vi "mockbusTesting.vi"() -> ()   [LabVIEW 2016]
uses:
  Common_FPGA_HealthAndStatus/DataTypes/HealthAndStatusSettings.ctl
  Common_FPGA_Modbus/DataTypes/ModbusPortSettings.ctl
  Common_FPGA_Timestamp/DataTypes/TimestampSettings.ctl
  FPGAMockHPILC/DataTypes/MockHPILCSettings.ctl
  <vilib>/rvi/Emulation/niFpgaGetClockAttributes.vi
  <vilib>/rvi/Emulation/niFpgaSctlEmulationGetInTimedLoop.vi
  <vilib>/rvi/Emulation/niFpgaEmulationReportErrorSimple.vi
  <vilib>/rvi/eio/common/nirviEmuTemplateMethod_errors.vi
  <vilib>/rvi/Emulation/niFpgaCriticalErrorInLSC.vi
  <vilib>/rvi/Emulation/niFpgaEmulationIsFPGAContextNoSignature.vi
  <vilib>/rvi/DataTransferAndStorage/Container/Common/niFpgaContainerGetUniqueNameForEmu.vi
  <vilib>/rvi/Memory/Memory_Emulation/niFpgaMemoryEmulationCacheClearOnFirstRun.vi
  <vilib>/rvi/Memory/Memory_Emulation/nirvimemoryEmulationManagerCache_MakeExclusive.vi
  <vilib>/rvi/Memory/Memory_Emulation/niFpgaMemoryEmulationValidateCache.vi
  <vilib>/rvi/Memory/Memory_Emulation/nirvimemoryEmulationManagerCache_InsertValue.vi
  <vilib>/Utility/error.llb/Clear Errors.vi
  <vilib>/rvi/Memory/Memory_Emulation/nirvimemoryEmulationManagerCache_ReleaseExclusive.vi
  <vilib>/rvi/Memory/Memory_Emulation/nirvimemoryEmulationManagerCache_GetValue.vi
  <vilib>/rvi/Memory/Memory_Emulation/nirvimemoryEmulationManagerCache_SetValue.vi
  <vilib>/rvi/Emulation/niFpgaProcessEmulError.vi
  <vilib>/eio/EIOMethodNode/EIOMethodNode.xnode
  <vilib>/rvi/DataTransferAndStorage/Container/XNode/niFpgaContainer.xnode
  <vilib>/rvi/DataTransferAndStorage/Register/Emulation/niFpgaRegisterEmulation.vi
  Common_FPGA_HealthAndStatus/FPGAHealthAndStatus.lvlib
  Common_FPGA_Modbus/FPGAModbus.lvlib
  Common_FPGA_Timestamp/FPGATimestamp.lvlib
  FPGAMockHPILC/FPGAMockHPILC.lvlib
panel:
  in  "Trigger":bool
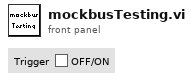
[diagram p1: front panel]
types:
  T1 = typedef "FPGAMockHPILC.lvlib/MockHPILCSettings.ctl" = cluster{"ModbusRxDataFIFO":refnum<k21>, "ModbusTxDataFIFO":refnum<k21>, "BufferUpdateFIFO":refnum<k21>, "Code17Memory":refnum<k21>, "Code18Memory":refnum<k21>, "Code65Memory":refnum<k21>, "Code66Memory":refnum<k21>, "Code67Memory":refnum<k21>, "Code72Memory":refnum<k21>, "Code80Memory":refnum<k21>, "Code110Memory":refnum<k21>, "CRCDataFIFO":refnum<k21>, "CRCCalculateFIFO":refnum<k21>, "CRCFIFO":refnum<k21>}
  T2 = typedef "FPGAModbus.lvlib/ModbusPortSettings.ctl" = cluster{"TxPort":refnum<k21>, "TxDataFIFO":refnum<k21>, "TxInternalDataFIFO":refnum<k21>, "TxHealthAndStatusFIFO":refnum<k21>, "RxPort":refnum<k21>, "RxDataFIFO":refnum<k21>, "RxHealthAndStatusFIFO":refnum<k21>, "BaseHealthAndStatusAddress":u32, "WaitForRxFrameRegister":refnum<k21>, "IRQAddress":u8, "TriggerIRQRegister":refnum<k21>, "InternalHealthAndStatusFIFO":refnum<k21>, "SoftwareControlledTrigger":refnum<k21>, "TimestampRegister":refnum<k21>, "TxTimestampFIFO":refnum<k21>}
  T3 = typedef "FPGATimestamp.lvlib/TimestampSettings.ctl" = cluster{"TimeRegister":refnum<k21>, "TimeSource":refnum<k21>, "IterationsPerMicrosecond":i16, "UpdateFIFO":refnum<k21>}
  T4 = typedef "FPGAHealthAndStatus.lvlib/HealthAndStatusSettings.ctl" = cluster{"InternalHealthAndStatusFIFO":refnum<k21>, "HealthAndStatusQueryFIFO":refnum<k21>, "HealthAndStatusResponseFIFO":refnum<k21>, "HealthAndStatusMemory":refnum<k21>, "MemorySize":i32}
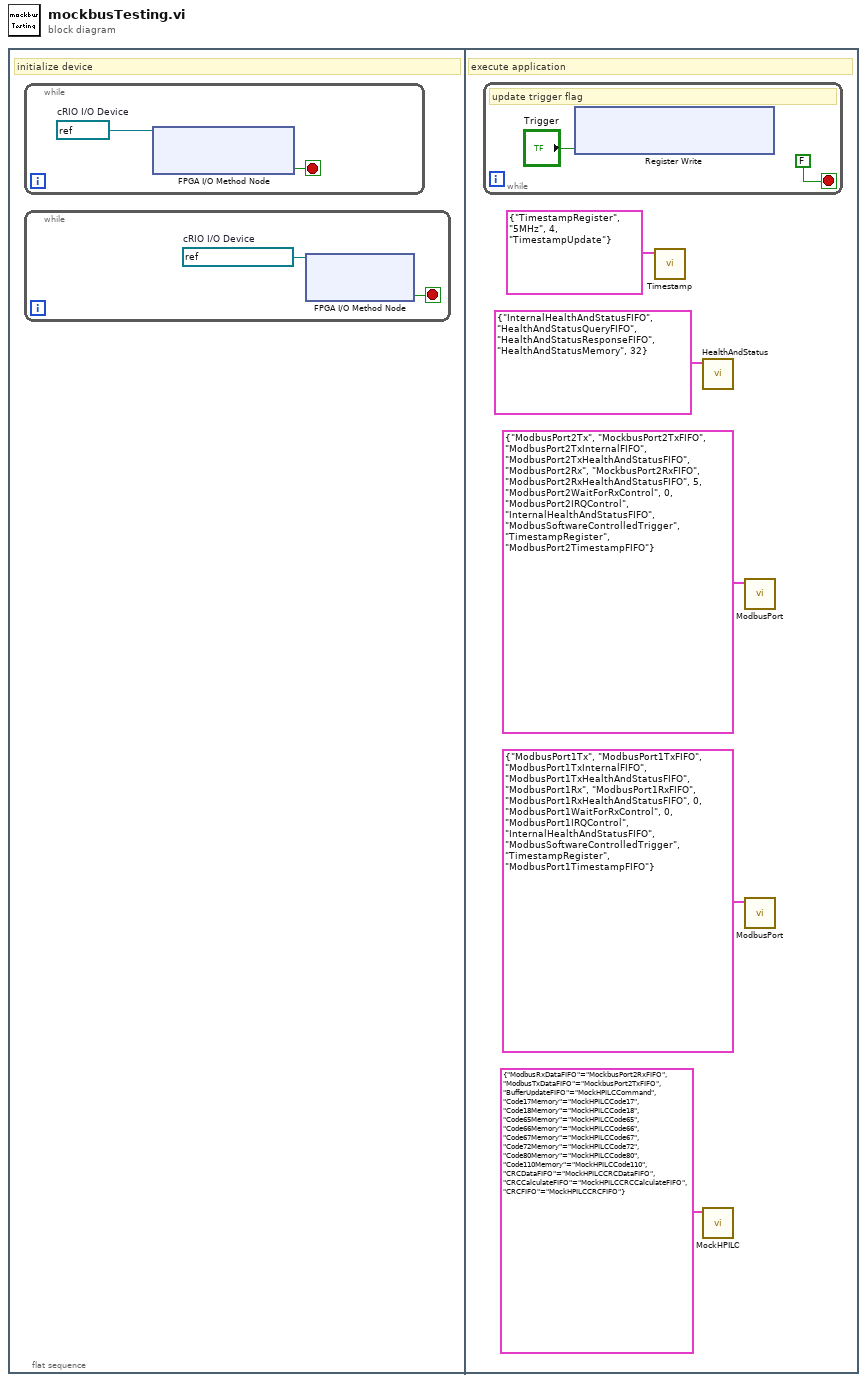
[diagram p0: block diagram]
diagram:
  n1 = flat-sequence {
    frame #0 {
      # "initialize device"
      n2 = while {
        stop <- w1 stop-if-true
        w2 = refnum<k21> "Sync"  # cRIO I/O Device
        n3 = xnode "FPGA I/O Method Node"("FPGA I/O In"=w2) -> ("Clock Running"=w1:bool)  [unwired: 1 out]
      }
      n4 = while {
        stop <- w3 stop-if-true
        w4 = refnum<k21> "ModbusPort1-4"  # cRIO I/O Device
        n5 = xnode "FPGA I/O Method Node"("FPGA I/O In"=w4) -> ("Ready"=w3:bool)  [unwired: 1 out]
      }
    }
    frame #1 {
      # "execute application"
      n6 = while {
        stop <- FALSE stop-if-true
        # "update trigger flag"
        n7 = xnode ("Register Write")("Data"="Trigger") -> ()  [unwired: 1 in, 1 out]
      }
      n8 = call "Timestamp.vi"("TimestampSettings"=T3 {"TimeRegister"="TimestampRegister", "TimeSource"="5MHz", "IterationsPerMicrosecond"=4, "UpdateFIFO"="TimestampUpdate"}) -> ()  [unwired: 11 in]
      n9 = call "HealthAndStatus.vi"("HealthAndStatusSettings"=T4 {"InternalHealthAndStatusFIFO"="InternalHealthAndStatusFIFO", "HealthAndStatusQueryFIFO"="HealthAndStatusQueryFIFO", "HealthAndStatusResponseFIFO"="HealthAndStatusResponseFIFO", "HealthAndStatusMemory"="HealthAndStatusMemory", "MemorySize"=32}) -> ()  [unwired: 11 in]
      n10 = call "MockHPILC.vi"("MockHPILCSettings"=T1 {"ModbusRxDataFIFO"="MockbusPort2RxFIFO", "ModbusTxDataFIFO"="MockbusPort2TxFIFO", "BufferUpdateFIFO"="MockHPILCCommand", "Code17Memory"="MockHPILCCode17", "Code18Memory"="MockHPILCCode18", "Code65Memory"="MockHPILCCode65", "Code66Memory"="MockHPILCCode66", "Code67Memory"="MockHPILCCode67", "Code72Memory"="MockHPILCCode72", "Code80Memory"="MockHPILCCode80", "Code110Memory"="MockHPILCCode110", "CRCDataFIFO"="MockHPILCCRCDataFIFO", "CRCCalculateFIFO"="MockHPILCCRCCalculateFIFO", "CRCFIFO"="MockHPILCCRCFIFO"}) -> ()  [unwired: 11 in]
      n11 = call "ModbusPort.vi"("ModbusPortSettings"=T2 {"TxPort"="ModbusPort2Tx", "TxDataFIFO"="MockbusPort2TxFIFO", "TxInternalDataFIFO"="ModbusPort2TxInternalFIFO", "TxHealthAndStatusFIFO"="ModbusPort2TxHealthAndStatusFIFO", "RxPort"="ModbusPort2Rx", "RxDataFIFO"="MockbusPort2RxFIFO", "RxHealthAndStatusFIFO"="ModbusPort2RxHealthAndStatusFIFO", "BaseHealthAndStatusAddress"=5, "WaitForRxFrameRegister"="ModbusPort2WaitForRxControl", "IRQAddress"=0, "TriggerIRQRegister"="ModbusPort2IRQControl", "InternalHealthAndStatusFIFO"="InternalHealthAndStatusFIFO", "SoftwareControlledTrigger"="ModbusSoftwareControlledTrigger", "TimestampRegister"="TimestampRegister", "TxTimestampFIFO"="ModbusPort2TimestampFIFO"}) -> ()  [unwired: 10 in]
      n12 = call "ModbusPort.vi"("ModbusPortSettings"=T2 {"TxPort"="ModbusPort1Tx", "TxDataFIFO"="ModbusPort1TxFIFO", "TxInternalDataFIFO"="ModbusPort1TxInternalFIFO", "TxHealthAndStatusFIFO"="ModbusPort1TxHealthAndStatusFIFO", "RxPort"="ModbusPort1Rx", "RxDataFIFO"="ModbusPort1RxFIFO", "RxHealthAndStatusFIFO"="ModbusPort1RxHealthAndStatusFIFO", "BaseHealthAndStatusAddress"=0, "WaitForRxFrameRegister"="ModbusPort1WaitForRxControl", "IRQAddress"=0, "TriggerIRQRegister"="ModbusPort1IRQControl", "InternalHealthAndStatusFIFO"="InternalHealthAndStatusFIFO", "SoftwareControlledTrigger"="ModbusSoftwareControlledTrigger", "TimestampRegister"="TimestampRegister", "TxTimestampFIFO"="ModbusPort1TimestampFIFO"}) -> ()  [unwired: 10 in]
    }
  }
